vi "Write String.vi"(7 "key":string, 8 "error in (no error)":errorcluster, 9 "default value":string, 10 "refnum":T1, 11 "Process in":refnum<class "Process.lvclass">) -> (0 "error out":errorcluster, 2 "refnum out":T1, 3 "Process out":refnum<class "Process.lvclass">)   [LabVIEW 2020, in "Configuration File.lvlib"]
doc: "High-level function for writing configuration file data from process class."
uses:
  Configuration File.lvlib
  User Interface/Process/Process.lvclass
  <vilib>/Utility/config.llb/NI_LVConfig.lvlib
  <vilib>/Utility/config.llb/Write Key (String).vi
  <vilib>/Utility/config.llb/Config Data RefNum.ctl
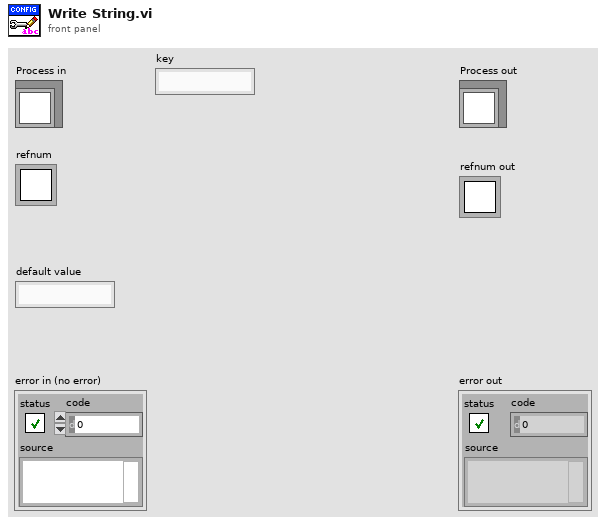
[diagram p1: front panel]
types:
  T1 = typedef "NI_LVConfig.lvlib/Config Data RefNum.ctl" = refnum<k1>
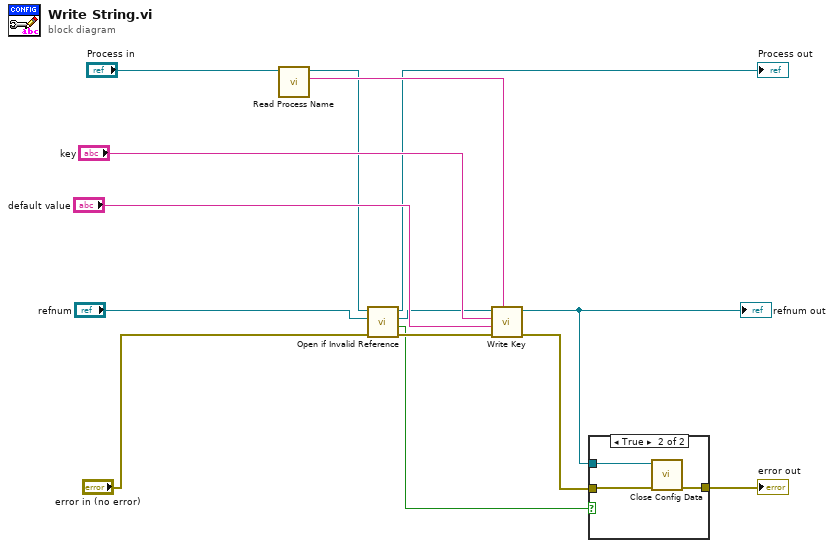
[diagram p0: block diagram]
diagram:
  n1 = call "Read Process Name.vi"("Process In"="Process in") -> ("Process Name"=w11:string, "Process Out"=w10:refnum<class "Process.lvclass">)  [unwired: 9 in]
  n2 = call "Open if Invalid Reference.vi"("error in (no error)"="error in (no error)", "refnum"="refnum", "Process in"=w10) -> ("error out"=w8:errorcluster, "File opened?"=w2:bool, "refnum out"=w6:T1, "Process out"=→"Process out":refnum<class "Process.lvclass">)  [unwired: 5 in]
  n3 = call-poly <vilib>:"Write Key.vi"("section"=w11, "error in (no error)"=w8, "value"="default value", "key"="key", "refnum"=w6) -> ("error out"=w5:errorcluster, "refnum out"=w3:T1)  [unwired: 4 in, 1 out]
  "refnum out" <- w3
  n4 = case shown="True" w2 {
    tunnel: w3 -> [_ w18]
    tunnel: w5 -> [w15 w17]
    tunnel: [w15 w16] -> w4
    frame False {
    }
    frame True {
      n5 = call <vilib>:"Close Config Data.vi"("error in (no error)"=w17, "refnum"=w18) -> ("error out"=w16:errorcluster)  [unwired: 8 in, 1 out]
    }
  }
  "error out" <- w4
